vi "Test Serialize Floating Point.vi"(8 "error in (no error)":errorcluster) -> (0 "error out":errorcluster)   [LabVIEW 2013]
uses:
  src/Serializer/JSON Serializer/JSON Serializer.lvclass
  <vilib>/addons/_JKI Toolkits/Caraya/classes/Test/Test.lvclass
  <vilib>/addons/_JKI Toolkits/Caraya/classes/Assert/Assert.lvclass
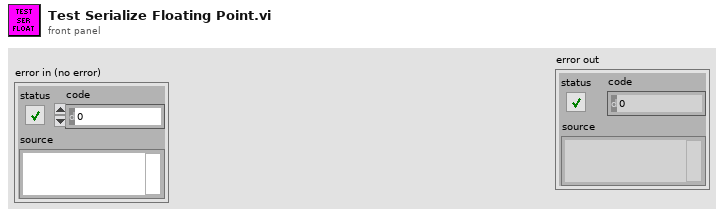
[diagram p1: front panel]
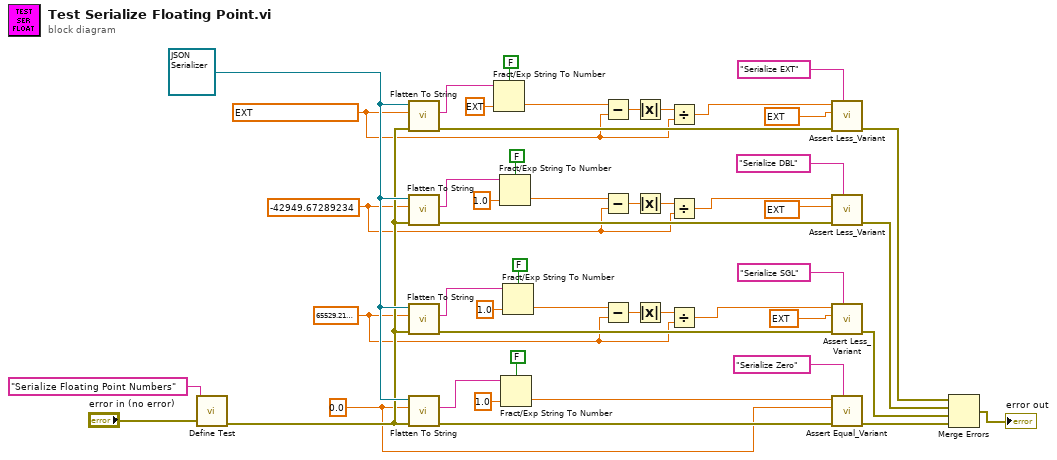
[diagram p0: block diagram]
diagram:
  w40 = refnum<class "JSON Serializer.lvclass"> refnum ("JKI JSON Serialization.lvlib:JSON Serializer.lvclass")
  w29 = 0.0
  w11 = ext 18446744073709551609.0
  w7 = sgl 65529.21
  w9 = -42949.67289234
  n1 = call <vilib>:"Define Test.vi"("error in (no error)"="error in (no error)", "Label (VI Title)"="Serialize Floating Point Numbers") -> ("error out"=w39:errorcluster)  [unwired: 9 in]
  n2 = call-dynamic "Flatten To String.vi"("error in (no error)"=w39, "Variant"=w11, "JSON Serializer in"=w40) -> ("error out"=w42:errorcluster, "String"=w19:string)  [unwired: 6 in, 1 out]
  n3 = call-dynamic "Flatten To String.vi"("error in (no error)"=w39, "Variant"=w9, "JSON Serializer in"=w40) -> ("error out"=w44:errorcluster, "String"=w22:string)  [unwired: 6 in, 1 out]
  n4 = call-dynamic "Flatten To String.vi"("error in (no error)"=w39, "Variant"=w7, "JSON Serializer in"=w40) -> ("error out"=w46:errorcluster, "String"=w25:string)  [unwired: 6 in, 1 out]
  n5 = call-dynamic "Flatten To String.vi"("error in (no error)"=w39, "Variant"=w29, "JSON Serializer in"=w40) -> ("error out"=w48:errorcluster, "String"=w32:string)  [unwired: 6 in, 1 out]
  n6 = Fract/Exp String To Number(use system decimal point (T)=FALSE, string=w19, default (0 dbl)=ext 1.0 ("default (0 DBL)")) -> (number=w17:ext)  [unwired: 1 in, 1 out]
  n7 = Fract/Exp String To Number(use system decimal point (T)=FALSE, string=w22, default (0 dbl)=1.0 ("default (0 DBL)")) -> (number=w18:dbl)  [unwired: 1 in, 1 out]
  n8 = Fract/Exp String To Number(use system decimal point (T)=FALSE, string=w32, default (0 dbl)=1.0 ("default (0 DBL)")) -> (number=w28:dbl)  [unwired: 1 in, 1 out]
  n9 = Fract/Exp String To Number(use system decimal point (T)=FALSE, string=w25, default (0 dbl)=sgl 1.0 ("default (0 DBL)")) -> (number=w16:sgl)  [unwired: 1 in, 1 out]
  n10 = Subtract(x=w17, y=w11) -> (x-y=w15:ext)
  n11 = Subtract(x=w18, y=w9) -> (x-y=w14:dbl)
  n12 = Subtract(x=w16, y=w7) -> (x-y=w13:sgl)
  n13 = Absolute Value(x=w15) -> (abs(x)=w12:ext)
  n14 = Absolute Value(x=w14) -> (abs(x)=w10:dbl)
  n15 = Absolute Value(x=w13) -> (abs(x)=w8:sgl)
  n16 = Divide(x=w12, y=w11) -> (x/y=w6:ext)
  n17 = Divide(x=w10, y=w9) -> (x/y=w5:dbl)
  n18 = Divide(x=w8, y=w7) -> (x/y=w4:sgl)
  n19 = call <vilib>:"Assert Less_Variant.vi"("Label"="Serialize EXT", "error in (no error)"=w42, "Y"=ext 1e-13 ("default (0 DBL)"), "X"=w6) -> ("error out"=w34:errorcluster)  [unwired: 7 in]
  n20 = call <vilib>:"Assert Less_Variant.vi"("Label"="Serialize DBL", "error in (no error)"=w44, "Y"=ext 1e-13 ("default (0 DBL)"), "X"=w5) -> ("error out"=w35:errorcluster)  [unwired: 7 in]
  n21 = call <vilib>:"Assert Less_Variant.vi"("Label"="Serialize SGL", "error in (no error)"=w46, "Y"=ext 0.00001 ("default (0 DBL)"), "X"=w4) -> ("error out"=w36:errorcluster)  [unwired: 7 in]
  n22 = call <vilib>:"Assert Equal_Variant.vi"("Label"="Serialize Zero", "error in (no error)"=w48, "Y"=w29, "X"=w28) -> ("error out"=w37:errorcluster)  [unwired: 7 in]
  n23 = Merge Errors(w34, w35, w36, w37) -> (→"error out":errorcluster)
